vi "E7_20.vi"(4 "error in":T13, 7 "Command":T14) -> (0 "error out":T13, 3 "Response":T11)   [LabVIEW 2018]
uses:
  MOKO_LabViewLibrary/MokoLowLevel/MokoLowLovelControl/MLLC_Command.ctl
  MOKO_LabViewLibrary/MokoLowLevel/MokoLowLovelControl/MLLC_Error.ctl
  MOKO_LabViewLibrary/MokoLowLevel/MokoLowLovelControl/MLLC_Mode.ctl
  MOKO_LabViewLibrary/MokoLowLevel/MokoLowLovelControl/MLLC_Response.ctl
  MOKO_LabViewLibrary/MokoLowLevel/MokoLowLovelControl/MLLC_DriverName.ctl
  MOKO_LabViewLibrary/MokoLowLevel/MokoLowLovelControl/MLLC_ResponseInit.ctl
  MOKO_LabViewLibrary/MokoLowLevel/MokoLowLovelControl/MLLC_ErrorCode.ctl
  MOKO_LabViewLibrary/MokoLowLevel/MokoLowLovelControl/MLLC_Request.ctl
  MOKO_LabViewLibrary/MokoLowLevel/MokoLowLovelControl/MLLC_ConnectCluster.ctl
  MOKO_LabViewLibrary/MokoLowLevel/MokoLowLovelControl/MLLC_InterfaceType.ctl
  MOKO_LabViewLibrary/MokoLowLevel/MokoLowLovelControl/MLLC_OpenedSession.ctl
  MOKO_LabViewLibrary/MokoLowLevel/MokoLowLovelControl/MLLC_InterfaceSettings.ctl
  MOKO_LabViewLibrary/MokoLowLevel/MokoLowLovelControl/MLLC_InterfaceKind.ctl
  MOKO_LabViewLibrary/MokoLowLevel/MokoLowLovelControl/MLLC_Rs232Settings.ctl
panel:
  in  "Settings":T7={"Data"={"Connect"={"InterfaceType"=enum."VISA", "OpenedSession"="", "InterfaceSettings"={"Interface"=enum."RS232", "EOS 4 read"=enum."LF (\\n)", "EOS 4 write"=enum."LF (\\n)", "TMO, ms"=10000, "Sett"=variant(cluster{"Baud Rate":u32, "Data Bits":u16, "Parity":u16, "Stop Bits":u16, "Flow Control":u16, "Eho":bool} {"Baud Rate"=75, "Data Bits"=0, "Parity"=0, "Stop Bits"=0, "Flow Control"=0, "Eho"=FALSE})}}, "Function"=enum."VDC", "Delay, ms"=100}, "Saved Data"=variant}
  in  "Request":T8
  in  "Error Code":T6=5422
  in  "ResponseInit":T9="Є"
  in  "Driver Name":T10="E7_20"
  in  "Mode":T12=enum."Check"
  # "E7-20"
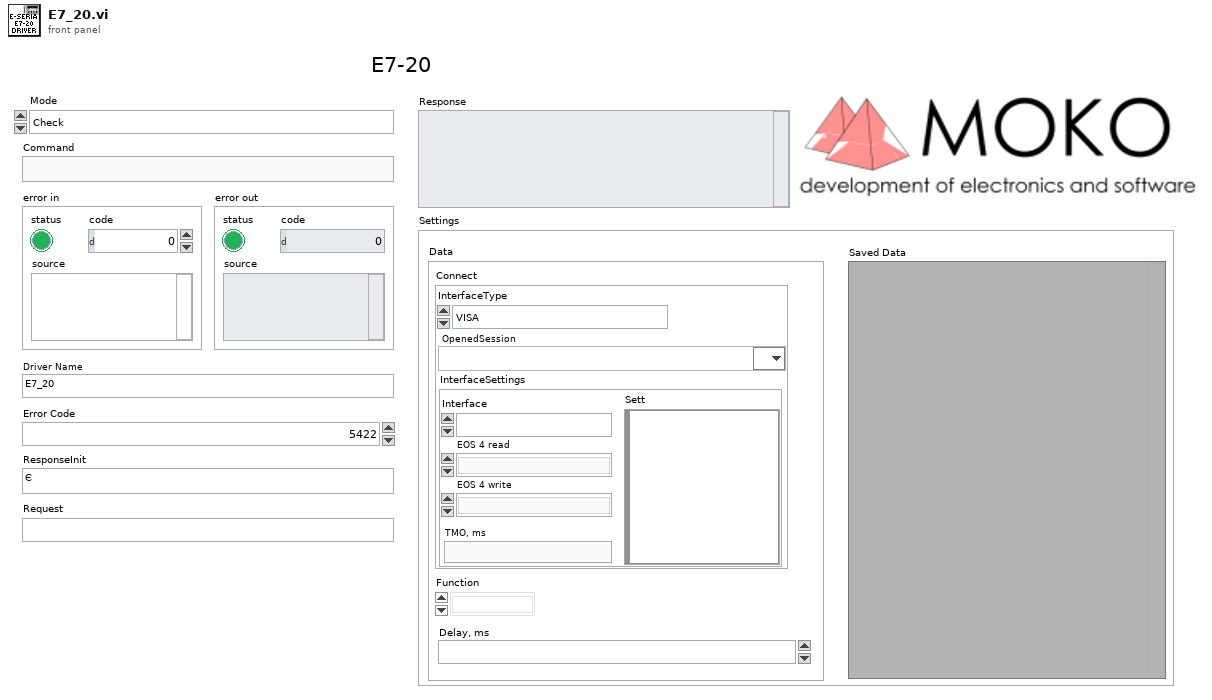
[diagram p1: front panel]
types:
  T1 = typedef "MLLC_ConnectCluster.ctl" = cluster{"InterfaceType":T2, "OpenedSession":T3, "InterfaceSettings":T4}
  T2 = typedef "MLLC_InterfaceType.ctl" = enum16{"VISA", "Prologix USB-GPIB"}
  T3 = typedef "MLLC_OpenedSession.ctl" = refnum<visa-resource-name>
  T4 = typedef "MLLC_InterfaceSettings.ctl" = cluster{"Interface":T5, "EOS 4 read":enum16{"Default (=EOS 4 write)", "CR (\\r)", "LF (\\n)", "None"}, "EOS 4 write":enum16{"CR+LF (\\r\\n)", "CR (\\r)", "LF (\\n)", "None"}, "TMO, ms":i32, "Sett":variant}
  T5 = typedef "MLLC_InterfaceKind.ctl" = enum16{"RS232", "GPIB", "USB", "Ethernet", "another"}
  T6 = typedef "MLLC_ErrorCode.ctl" = u32
  T7 = cluster{"Data":cluster{"Connect":T1, "Function":enum16{"F", "T", "R4", "R", "IAC", "IDC", "VAC", "VDC"}, "Delay, ms":T6}, "Saved Data":variant}
  T8 = typedef "MLLC_Request.ctl" = string
  T9 = typedef "MLLC_ResponseInit.ctl" = string
  T10 = typedef "MLLC_DriverName.ctl" = string
  T11 = typedef "MLLC_Response.ctl" = string
  T12 = typedef "MLLC_Mode.ctl" = enum16{"get", "set", "close", "Init", "Check"}
  T13 = typedef "MLLC_Error.ctl" = errorcluster
  T14 = typedef "MLLC_Command.ctl" = string
  T15 = cluster{"Connect":T1, "Function":enum16{"F", "T", "R4", "R", "IAC", "IDC", "VAC", "VDC"}, "Delay, ms":T6}
  T16 = typedef "MLLC_Rs232Settings.ctl" = cluster{"Baud Rate":u32, "Data Bits":u16, "Parity":u16, "Stop Bits":u16, "Flow Control":u16, "Eho":bool, "Address":dbl}
  T17 = enum16{"F", "T", "R4", "R", "IAC", "IDC", "VAC", "VDC"}
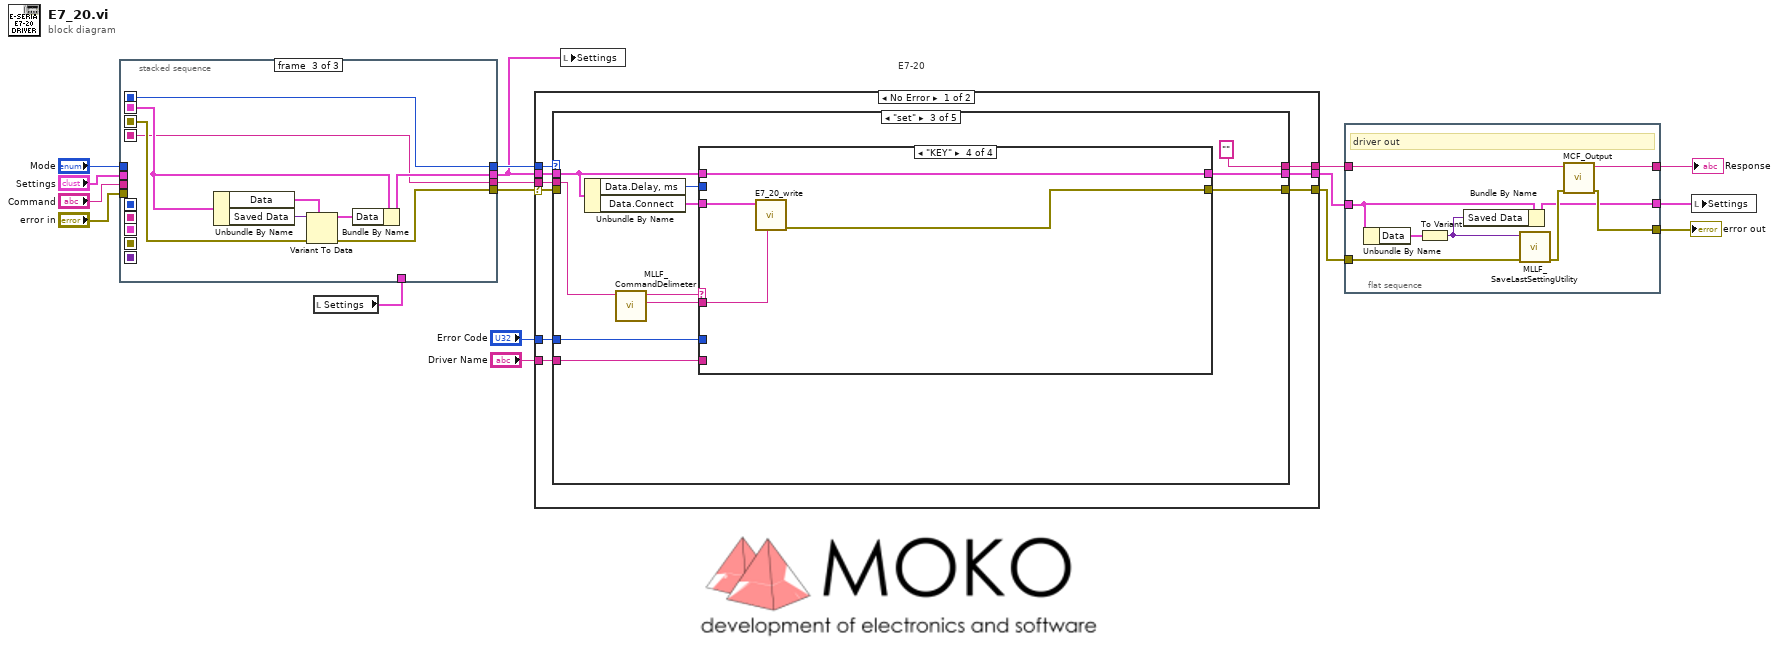
[diagram p0: block diagram]
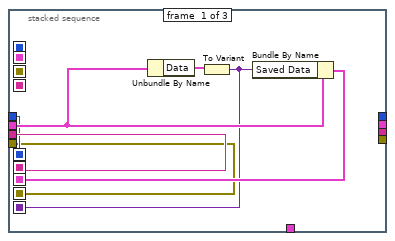
[diagram p2: hidden frame]
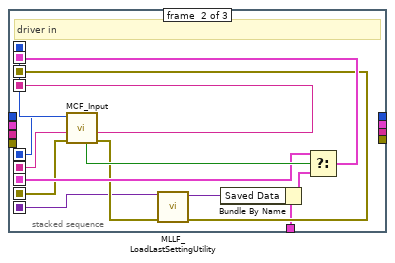
[diagram p3: hidden frame]
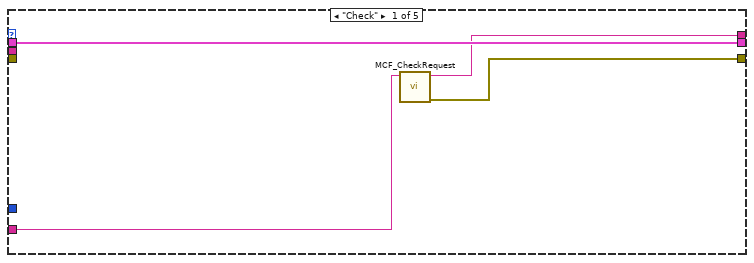
[diagram p4: hidden frame]
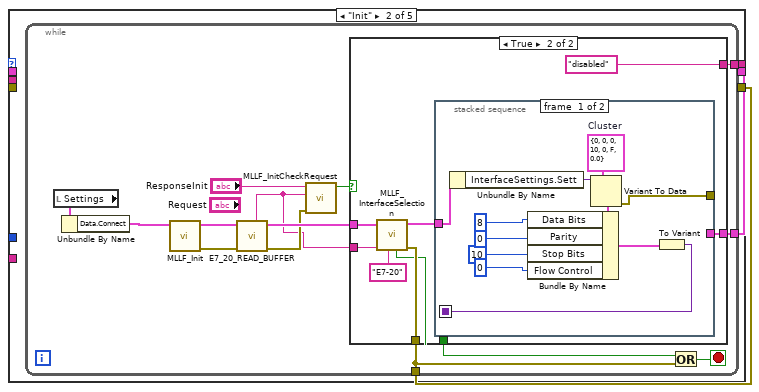
[diagram p5: hidden frame]
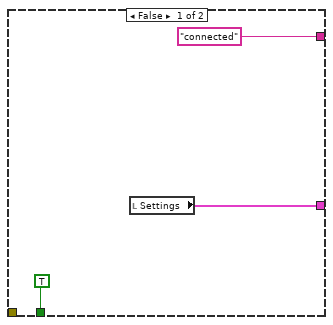
[diagram p6: hidden frame]
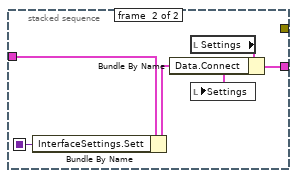
[diagram p7: hidden frame]
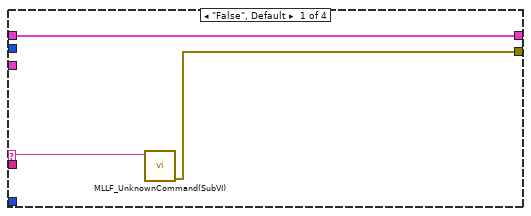
[diagram p8: hidden frame]
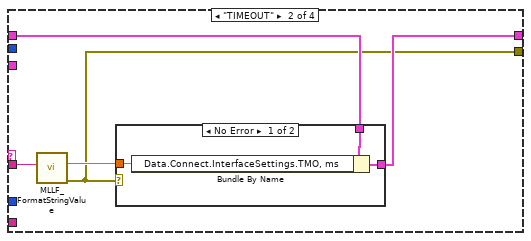
[diagram p9: hidden frame]
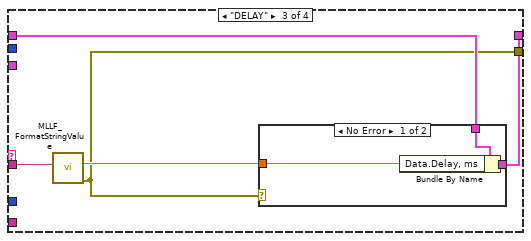
[diagram p11: hidden frame]
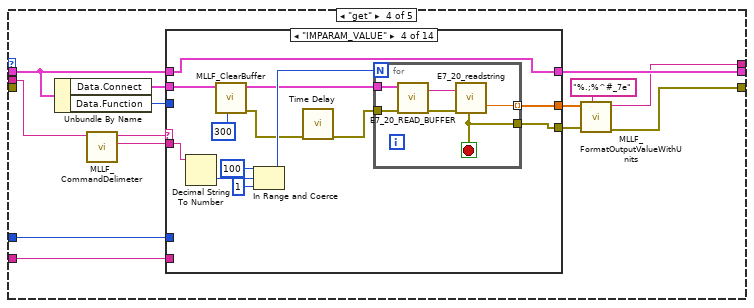
[diagram p13: hidden frame]
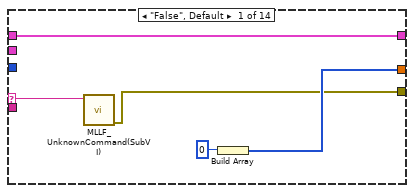
[diagram p14: hidden frame]
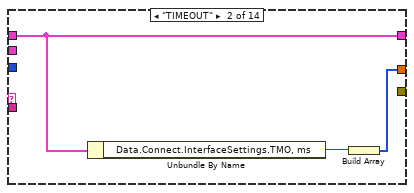
[diagram p15: hidden frame]
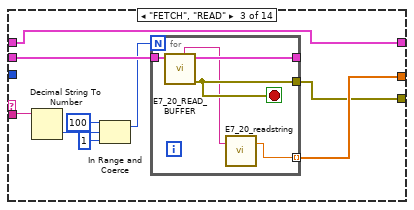
[diagram p16: hidden frame]
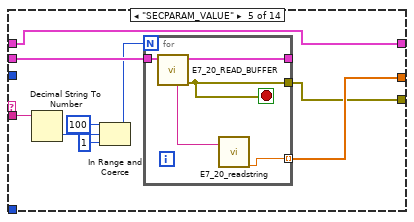
[diagram p17: hidden frame]
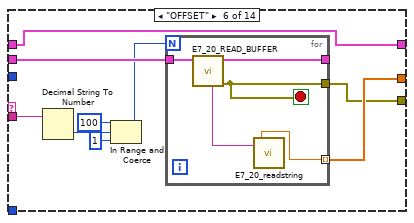
[diagram p18: hidden frame]
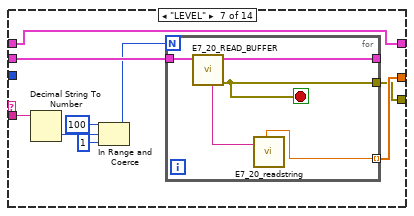
[diagram p19: hidden frame]
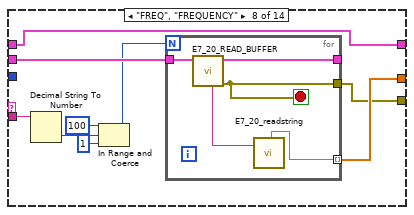
[diagram p20: hidden frame]
diagram:
  # "E7-20"
  n1 = local read "Settings"() -> (w7:T7)
  n2 = stacked-sequence {
    seq-local: [w20 _ _] -> [_ w36 _]
    seq-local: [w19 _ _] -> [_ w37 _]
    seq-local: [w22 _ _] -> [_ w32 _]
    seq-local: [w18 _ _] -> [_ w31 _]
    seq-local: [w21 _ _] -> [_ w27 _]
    seq-local: [_ w28 _] -> [_ _ w44]
    seq-local: [_ w38 _] -> [_ _ w41]
    seq-local: [_ w35 _] -> [_ _ w40]
    seq-local: [_ w34 _] -> [_ _ w45]
    tunnel: "Command" -> [w20 _ _]
    tunnel: "Mode" -> [w19 _ _]
    tunnel: "error in" -> [w18 _ _]
    tunnel: "Settings" -> [w23 _ _]
    tunnel: w7 -> [_ w26 _]
    tunnel: [_ _ w40] -> w9
    tunnel: [_ _ w43] -> w10
    tunnel: [_ _ w42] -> w8
    tunnel: [_ _ w41] -> w11
    frame #0 {
      n3 = Unbundle By Name(w23) -> ("Data"=w24:T15)
      n4 = To Variant(anything=w24) -> (Variant=w21:variant)
      n5 = Bundle By Name(cluster=w23, "Saved Data"=w21) -> (w22:T7)
    }
    frame #1 {
      # "driver in"
      n6 = call "MCF_Input.vi"("Error In"=w31, "Command in"=w36, "Mode in"=w37) -> ("Error Out"=w30:errorcluster, "Command out"=w35:string, "Mode out"=w38:T12, "Boolean"=w33:bool)  [unwired: 5 in]
      n7 = call "MLLF_LoadLastSettingUtility.vi"("Error In"=w30, "Save data in"=w27) -> ("Error Out"=w28:errorcluster, "Save data out"=w25:variant)  [unwired: 8 in]
      n8 = Bundle By Name(cluster=w26, "Saved Data"=w25) -> (w29:T7)
      n9 = Select(t=w32, s=w33, f=w29) -> (s? t:f=w34:T7)
    }
    frame #2 {
      n10 = Unbundle By Name(w45) -> ("Data"=w46:T15, "Saved Data"=w39:variant)
      n11 = Variant To Data(error in=w44, type=w46, Variant=w39) -> (data=w47:T15, error out=w42:errorcluster)
      n12 = Bundle By Name(cluster=w45, "Data"=w47) -> (w43:T7)
    }
  }
  n13 = case shown="No Error" w8 {
    selector: w8 -> [w52 w341]
    tunnel: [w54 w341] -> w4
    tunnel: w11 -> [w56 _]
    tunnel: [w55 "" ("String")] -> w6
    tunnel: w9 -> [w53 _]
    tunnel: w10 -> [w49 w340]
    tunnel: "Error Code" -> [w51 _]
    tunnel: "Driver Name" -> [w50 _]
    tunnel: [w48 w340] -> w5
    frame No Error {
      n14 = case shown="\"set\"" w56 {
        tunnel: [w59 w63 "" ("String") w141 _] -> w55
        tunnel: [w58 w61 w105 w142 w337] -> w54
        tunnel: w53 -> [_ _ w108 w145 _]
        tunnel: w52 -> [_ _ _ _ _]
        tunnel: w51 -> [_ _ w115 w152 _]
        tunnel: w50 -> [w57 _ w112 w151 _]
        tunnel: w49 -> [w60 _ w114 w154 w336]
        tunnel: [w60 w62 w113 w153 w336] -> w48
        frame "Check" {
          n15 = call "MCF_CheckRequest.vi"("Driver Name"=w57) -> ("Error Out"=w58:errorcluster, "Output String"=w59:string)  [unwired: 9 in]
        }
        frame "Init" {
          n16 = while {
            tunnel: [w75] -> w61
            tunnel: [w66] -> w63
            tunnel: [w65] -> w62
            stop <- w74 stop-if-true
            n17 = local read "Settings"() -> (w77:T7)
            n18 = Unbundle By Name(w77) -> ("Data.Connect"=w76:T1)
            n19 = call "MLLF_Init.vi"("DriverConnect in"=w76) -> ("Error Out"=w70:errorcluster, "DriverConnect out"=w71:T1)  [unwired: 7 in]
            n20 = call "E7_20_READ_BUFFER.vi"("error in"=w70, "DriverConnect in"=w71) -> ("error out"=w68:T13, "DriverConnect out"=w72:T1, "String"=w64:string)  [unwired: 7 in]
            n21 = call "MLLF_InitCheckRequest.vi"("error in (no error)"=w68, "Answer"=w64, "Response Init"="ResponseInit") -> ("Design"=w67:bool)  [unwired: 5 in, 3 out]
            n22 = case shown="True" w67 {
              tunnel: [_ w86] -> w75
              tunnel: [TRUE w82] -> w73
              tunnel: w72 -> [_ w88]
              tunnel: ["connected" "disabled"] -> w66
              tunnel: [w78 w83] -> w65
              tunnel: w64 -> [_ w81]
              frame False {
                n23 = local read "Settings"() -> (w78:T7)
              }
              frame True {
                n24 = call "MLLF_InterfaceSelection.vi"("Driver Name"="E7-20" ("String"), "Answer:"=w81, "DriverConnect in"=w88) -> ("error out"=w86:T13, "DriverConnect out"=w87:T1, "stop init?"=w82:bool)  [unwired: 4 in, 2 out]
                n25 = stacked-sequence {
                  seq-local: [w91 _] -> [_ w103]
                  tunnel: w87 -> [w89 w101]
                  tunnel: [w97 _] -> _
                  tunnel: [_ w102] -> w83
                  frame #0 {
                    w98 = T16 {"Baud Rate"=0, "Data Bits"=0, "Parity"=0, "Stop Bits"=10, "Flow Control"=0, "Eho"=FALSE, "Address"=0.0}  # Cluster
                    n26 = Unbundle By Name(w89) -> ("InterfaceSettings.Sett"=w99:variant)
                    n27 = Variant To Data(type=w98, Variant=w99) -> (data=w96:T16, error out=w97:errorcluster)  [unwired: 1 in]
                    n28 = Bundle By Name(cluster=w96, "Data Bits"=u16 8 ("Serial Settings:Data Bits"), "Parity"=u16 0 ("Serial Settings:Parity"), "Stop Bits"=u16 10 ("Serial Settings:Stop Bits"), "Flow Control"=u16 0 ("Serial Settings:Flow Control")) -> (w90:T16)
                    n29 = To Variant(anything=w90) -> (Variant=w91:variant)
                  }
                  frame #1 {
                    n30 = Bundle By Name(cluster=w101, "InterfaceSettings.Sett"=w103) -> (w100:T1)
                    n31 = local read "Settings"() -> (w104:T7)
                    n32 = Bundle By Name(cluster=w104, "Data.Connect"=w100) -> (w102:T7)
                    n33 = local write "Settings"(w102) -> ()
                  }
                }
              }
            }
            n34 = Or(x=w73, y=w75) -> (x .or. y?=w74:bool)
          }
        }
        frame "set" {
          n35 = Unbundle By Name(w114) -> ("Data.Delay, ms"=w109:T6, "Data.Connect"=w110:T1)
          n36 = call "MLLF_CommandDelimeter.vi"("command with param"=w108) -> ("param 1"=w106:string, "command"=w107:string)  [unwired: 6 in, 3 out]
          n37 = case shown="\"KEY\"" w107 {
            selector: w107 -> [w117 _ _ _]
            tunnel: w106 -> [_ w121 w130 w139]
            tunnel: [w116 w119 w128 w138] -> w105
            tunnel: w115 -> [_ _ _ _]
            tunnel: w114 -> [w118 w122 w131 w140]
            tunnel: [w118 w123 w132 w140] -> w113
            tunnel: w110 -> [_ _ _ w137]
            tunnel: w112 -> [_ _ _ _]
            tunnel: w109 -> [_ _ _ _]
            frame "False", Default {
              n38 = call "MLLF_UnknownCommand(SubVI).vi"("Unknown command"=w117) -> ("error out"=w116:errorcluster)  [unwired: 10 in]
            }
            frame "TIMEOUT" {
              n39 = call "MLLF_FormatStringValue.vi"("String Value"=w121) -> ("error out"=w119:T13, "number"=w120:dbl)  [unwired: 8 in, 1 out]
              n40 = case shown="No Error" w119 {
                tunnel: [w126 w127] -> w123
                tunnel: w122 -> [w125 w127]
                tunnel: w120 -> [w124 _]
                frame No Error {
                  n41 = Bundle By Name(cluster=w125, "Data.Connect.InterfaceSettings.TMO, ms"=w124) -> (w126:T7)
                }
                frame Error {
                }
              }
            }
            frame "DELAY" {
              n42 = call "MLLF_FormatStringValue.vi"("String Value"=w130) -> ("error out"=w128:T13, "number"=w129:dbl)  [unwired: 8 in, 1 out]
              n43 = case shown="No Error" w128 {
                tunnel: [w135 w136] -> w132
                tunnel: w131 -> [w134 w136]
                tunnel: w129 -> [w133 _]
                frame No Error {
                  n44 = Bundle By Name(cluster=w134, "Data.Delay, ms"=w133) -> (w135:T7)
                }
                frame Error {
                }
              }
            }
            frame "KEY" {
              n45 = call "E7_20_write.vi"("Command"=w139, "DriverConnect in"=w137) -> ("error out"=w138:T13)  [unwired: 8 in, 1 out]
            }
          }
        }
        frame "get" {
          n46 = Unbundle By Name(w154) -> ("Data.Connect"=w148:T1, "Data.Function"=w146:T17)
          n47 = call "MLLF_CommandDelimeter.vi"("command with param"=w145) -> ("param 1"=w143:string, "command"=w144:string)  [unwired: 6 in, 3 out]
          n48 = case shown="\"IMPARAM_VALUE\"" w144 {
            selector: w144 -> [w156 _ _ _ _ _ _ _ _ _ _ _ _ _]
            tunnel: w143 -> [_ _ w163 w177 w196 w210 w224 w238 w252 w266 w280 w294 w308 w322]
            tunnel: [w155 _ w168 w187 w201 w215 w229 w243 w257 w271 w285 w299 w313 w327] -> w150
            tunnel: w152 -> [_ _ _ _ _ _ _ _ _ _ _ _ _ _]
            tunnel: [w159 w162 w171 w189 w204 w218 w232 w246 w260 w274 w288 w302 w316 w330] -> w153
            tunnel: w154 -> [w159 w162 w171 w189 w204 w218 w232 w246 w260 w274 w288 w302 w316 w330]
            tunnel: [w157 w160 w169 w188 w202 w216 w230 w244 w258 w272 w286 w300 w314 w328] -> w149
            tunnel: w148 -> [_ _ w170 w180 w203 w217 w231 w245 w259 w273 w287 w301 w315 w329]
            tunnel: w151 -> [_ _ _ _ _ _ _ _ _ _ _ _ _ _]
            tunnel: w146 -> [_ _ _ _ _ _ _ _ _ _ _ _ _ _]
            frame "False", Default {
              n49 = call "MLLF_UnknownCommand(SubVI).vi"("Unknown command"=w156) -> ("error out"=w155:errorcluster)  [unwired: 10 in]
              n50 = Build Array(0 ("TimeOut")) -> (w157:i32[])
            }
            frame "TIMEOUT" {
              n51 = Unbundle By Name(w162) -> ("Data.Connect.InterfaceSettings.TMO, ms"=w161:i32)
              n52 = Build Array(w161) -> (w160:i32[])
            }
            frame "FETCH", "READ" {
              n53 = Decimal String To Number(string=w163) -> (number=w167:i32)  [unwired: 2 in, 1 out]
              n54 = In Range and Coerce(upper limit=100, x=w167, lower limit=1) -> (coerced(x)=w164:i32)  [unwired: 1 out]
              n55 = for {
                N: w164 -> [_]
                tunnel: [w172] -> w169 mode=indexing
                tunnel: [w175] -> w168
                tunnel: [w176] -> _
                tunnel: w170 -> [w174]
                stop <- w175 stop-if-true
                n56 = call "E7_20_READ_BUFFER.vi"("DriverConnect in"=w174) -> ("error out"=w175:T13, "DriverConnect out"=w176:T1, "String"=w173:string)  [unwired: 8 in]
                n57 = call "E7_20_readstring.vi"("read buffer"=w173) -> ("CS"=w172:dbl)  [unwired: 6 in, 12 out]
              }
            }
            frame "IMPARAM_VALUE" {
              n58 = Decimal String To Number(string=w177) -> (number=w186:i32)  [unwired: 2 in, 1 out]
              n59 = call "MLLF_ClearBuffer.vi"("Timeout(default = 300 ms)"=u32 300 ("Timeout"), "DriverConnect in"=w180) -> ("Error Out"=w179:errorcluster, "DriverConnect out"=w181:T1)  [unwired: 6 in, 1 out]
              n60 = In Range and Coerce(upper limit=100, x=w186, lower limit=1) -> (coerced(x)=w183:i32)  [unwired: 1 out]
              n61 = call "Time Delay"("error in (no error)"=w179) -> ("error out"=w178:errorcluster)  [unwired: 10 in]
              n62 = for {
                N: w183 -> [_]
                tunnel: [w193] -> w188 mode=indexing
                tunnel: [w191] -> w187
                tunnel: w181 -> [w194]
                tunnel: w178 -> [w190]
                stop <- w191 stop-if-true
                n63 = call "E7_20_READ_BUFFER.vi"("error in"=w190, "DriverConnect in"=w194) -> ("error out"=w192:T13, "String"=w195:string)  [unwired: 7 in, 1 out]
                n64 = call "E7_20_readstring.vi"("read buffer"=w195, "Error In"=w192) -> ("Error Out"=w191:errorcluster, "ImParam_Value"=w193:dbl)  [unwired: 5 in, 11 out]
              }
            }
            frame "SECPARAM_VALUE" {
              n65 = Decimal String To Number(string=w196) -> (number=w200:i32)  [unwired: 2 in, 1 out]
              n66 = In Range and Coerce(upper limit=100, x=w200, lower limit=1) -> (coerced(x)=w197:i32)  [unwired: 1 out]
              n67 = for {
                N: w197 -> [_]
                tunnel: [w205] -> w202 mode=indexing
                tunnel: [w208] -> w201
                tunnel: [w209] -> _
                tunnel: w203 -> [w206]
                stop <- w208 stop-if-true
                n68 = call "E7_20_READ_BUFFER.vi"("DriverConnect in"=w206) -> ("error out"=w208:T13, "DriverConnect out"=w209:T1, "String"=w207:string)  [unwired: 8 in]
                n69 = call "E7_20_readstring.vi"("read buffer"=w207) -> ("SecParam_Value"=w205:dbl)  [unwired: 6 in, 12 out]
              }
            }
            frame "OFFSET" {
              n70 = Decimal String To Number(string=w210) -> (number=w214:i32)  [unwired: 2 in, 1 out]
              n71 = In Range and Coerce(upper limit=100, x=w214, lower limit=1) -> (coerced(x)=w211:i32)  [unwired: 1 out]
              n72 = for {
                N: w211 -> [_]
                tunnel: [w219] -> w216 mode=indexing
                tunnel: [w222] -> w215
                tunnel: [w223] -> _
                tunnel: w217 -> [w220]
                stop <- w222 stop-if-true
                n73 = call "E7_20_READ_BUFFER.vi"("DriverConnect in"=w220) -> ("error out"=w222:T13, "DriverConnect out"=w223:T1, "String"=w221:string)  [unwired: 8 in]
                n74 = call "E7_20_readstring.vi"("read buffer"=w221) -> ("Offset"=w219:dbl)  [unwired: 6 in, 12 out]
              }
            }
            frame "LEVEL" {
              n75 = Decimal String To Number(string=w224) -> (number=w228:i32)  [unwired: 2 in, 1 out]
              n76 = In Range and Coerce(upper limit=100, x=w228, lower limit=1) -> (coerced(x)=w225:i32)  [unwired: 1 out]
              n77 = for {
                N: w225 -> [_]
                tunnel: [w233] -> w230 mode=indexing
                tunnel: [w236] -> w229
                tunnel: [w237] -> _
                tunnel: w231 -> [w234]
                stop <- w236 stop-if-true
                n78 = call "E7_20_READ_BUFFER.vi"("DriverConnect in"=w234) -> ("error out"=w236:T13, "DriverConnect out"=w237:T1, "String"=w235:string)  [unwired: 8 in]
                n79 = call "E7_20_readstring.vi"("read buffer"=w235) -> ("Level"=w233:dbl)  [unwired: 6 in, 12 out]
              }
            }
            frame "FREQ", "FREQUENCY" {
              n80 = Decimal String To Number(string=w238) -> (number=w242:i32)  [unwired: 2 in, 1 out]
              n81 = In Range and Coerce(upper limit=100, x=w242, lower limit=1) -> (coerced(x)=w239:i32)  [unwired: 1 out]
              n82 = for {
                N: w239 -> [_]
                tunnel: [w247] -> w244 mode=indexing
                tunnel: [w250] -> w243
                tunnel: [w251] -> _
                tunnel: w245 -> [w248]
                stop <- w250 stop-if-true
                n83 = call "E7_20_READ_BUFFER.vi"("DriverConnect in"=w248) -> ("error out"=w250:T13, "DriverConnect out"=w251:T1, "String"=w249:string)  [unwired: 8 in]
                n84 = call "E7_20_readstring.vi"("read buffer"=w249) -> ("Frequency"=w247:dbl)  [unwired: 6 in, 12 out]
              }
            }
            frame "FLAGS" {
              n85 = Decimal String To Number(string=w252) -> (number=w256:i32)  [unwired: 2 in, 1 out]
              n86 = In Range and Coerce(upper limit=100, x=w256, lower limit=1) -> (coerced(x)=w253:i32)  [unwired: 1 out]
              n87 = for {
                N: w253 -> [_]
                tunnel: [w261] -> w258 mode=indexing
                tunnel: [w264] -> w257
                tunnel: [w265] -> _
                tunnel: w259 -> [w262]
                stop <- w264 stop-if-true
                n88 = call "E7_20_READ_BUFFER.vi"("DriverConnect in"=w262) -> ("error out"=w264:T13, "DriverConnect out"=w265:T1, "String"=w263:string)  [unwired: 8 in]
                n89 = call "E7_20_readstring.vi"("read buffer"=w263) -> ("FLAGS"=w261:dbl)  [unwired: 6 in, 12 out]
              }
            }
            frame "MODE" {
              n90 = Decimal String To Number(string=w266) -> (number=w270:i32)  [unwired: 2 in, 1 out]
              n91 = In Range and Coerce(upper limit=100, x=w270, lower limit=1) -> (coerced(x)=w267:i32)  [unwired: 1 out]
              n92 = for {
                N: w267 -> [_]
                tunnel: [w275] -> w272 mode=indexing
                tunnel: [w278] -> w271
                tunnel: [w279] -> _
                tunnel: w273 -> [w276]
                stop <- w278 stop-if-true
                n93 = call "E7_20_READ_BUFFER.vi"("DriverConnect in"=w276) -> ("error out"=w278:T13, "DriverConnect out"=w279:T1, "String"=w277:string)  [unwired: 8 in]
                n94 = call "E7_20_readstring.vi"("read buffer"=w277) -> ("Mode"=w275:dbl)  [unwired: 6 in, 12 out]
              }
            }
            frame "LIMIT" {
              n95 = Decimal String To Number(string=w280) -> (number=w284:i32)  [unwired: 2 in, 1 out]
              n96 = In Range and Coerce(upper limit=100, x=w284, lower limit=1) -> (coerced(x)=w281:i32)  [unwired: 1 out]
              n97 = for {
                N: w281 -> [_]
                tunnel: [w289] -> w286 mode=indexing
                tunnel: [w292] -> w285
                tunnel: [w293] -> _
                tunnel: w287 -> [w290]
                stop <- w292 stop-if-true
                n98 = call "E7_20_READ_BUFFER.vi"("DriverConnect in"=w290) -> ("error out"=w292:T13, "DriverConnect out"=w293:T1, "String"=w291:string)  [unwired: 8 in]
                n99 = call "E7_20_readstring.vi"("read buffer"=w291) -> ("Limit"=w289:dbl)  [unwired: 6 in, 12 out]
              }
            }
            frame "IMPARAM" {
              n100 = Decimal String To Number(string=w294) -> (number=w298:i32)  [unwired: 2 in, 1 out]
              n101 = In Range and Coerce(upper limit=100, x=w298, lower limit=1) -> (coerced(x)=w295:i32)  [unwired: 1 out]
              n102 = for {
                N: w295 -> [_]
                tunnel: [w303] -> w300 mode=indexing
                tunnel: [w306] -> w299
                tunnel: [w307] -> _
                tunnel: w301 -> [w304]
                stop <- w306 stop-if-true
                n103 = call "E7_20_READ_BUFFER.vi"("DriverConnect in"=w304) -> ("error out"=w306:T13, "DriverConnect out"=w307:T1, "String"=w305:string)  [unwired: 8 in]
                n104 = call "E7_20_readstring.vi"("read buffer"=w305) -> ("ImParam"=w303:dbl)  [unwired: 6 in, 12 out]
              }
            }
            frame "SECPARAM" {
              n105 = Decimal String To Number(string=w308) -> (number=w312:i32)  [unwired: 2 in, 1 out]
              n106 = In Range and Coerce(upper limit=100, x=w312, lower limit=1) -> (coerced(x)=w309:i32)  [unwired: 1 out]
              n107 = for {
                N: w309 -> [_]
                tunnel: [w317] -> w314 mode=indexing
                tunnel: [w320] -> w313
                tunnel: [w321] -> _
                tunnel: w315 -> [w318]
                stop <- w320 stop-if-true
                n108 = call "E7_20_READ_BUFFER.vi"("DriverConnect in"=w318) -> ("error out"=w320:T13, "DriverConnect out"=w321:T1, "String"=w319:string)  [unwired: 8 in]
                n109 = call "E7_20_readstring.vi"("read buffer"=w319) -> ("SecParam"=w317:dbl)  [unwired: 6 in, 12 out]
              }
            }
            frame "ONCHANGE" {
              n110 = Decimal String To Number(string=w322) -> (number=w326:i32)  [unwired: 2 in, 1 out]
              n111 = In Range and Coerce(upper limit=100, x=w326, lower limit=1) -> (coerced(x)=w323:i32)  [unwired: 1 out]
              n112 = for {
                N: w323 -> [_]
                tunnel: [w331] -> w328 mode=indexing
                tunnel: [w334] -> w327
                tunnel: [w335] -> _
                tunnel: w329 -> [w332]
                stop <- w334 stop-if-true
                n113 = call "E7_20_READ_BUFFER.vi"("DriverConnect in"=w332) -> ("error out"=w334:T13, "DriverConnect out"=w335:T1, "String"=w333:string)  [unwired: 8 in]
                n114 = call "E7_20_readstring.vi"("read buffer"=w333) -> ("OnChange"=w331:dbl)  [unwired: 6 in, 12 out]
              }
            }
          }
          n115 = call "MLLF_FormatOutputValueWithUnits.vi"("Format"="%.;%^#_7e" ("format string"), "error in"=w150, "ValuesIn"=w149) -> ("error out"=w142:T13, "Result string"=w141:T14)  [unwired: 7 in]
        }
        frame "close" {
          n116 = Unbundle By Name(w336) -> ("Data.Connect.OpenedSession"=w338:T3)
          n117 = VISA Close(VISA resource name=w338) -> (error out=w337:errorcluster)  [unwired: 1 in]
        }
      }
    }
    frame Error {
    }
  }
  n118 = local write "Settings"(w10) -> ()
  n119 = flat-sequence {
    tunnel: [w350] -> w3
    tunnel: [w349] -> w1
    tunnel: w6 -> [w348]
    tunnel: w4 -> [w347]
    tunnel: w5 -> [w343]
    tunnel: [w345] -> w2
    frame #0 {
      # "driver out"
      n120 = Unbundle By Name(w343) -> ("Data"=w342:T15)
      n121 = To Variant(anything=w342) -> (Variant=w344:variant)
      n122 = Bundle By Name(cluster=w343, "Saved Data"=w344) -> (w345:T7)
      n123 = call "MLLF_SaveLastSettingUtility.vi"("error in"=w347, "Saved Data"=w344) -> ("error out"=w346:T13)  [unwired: 8 in, 1 out]
      n124 = call "MCF_Output.vi"("Error In"=w346, "Input"=w348) -> ("Error Out"=w349:errorcluster, "Output"=w350:string)  [unwired: 8 in]
    }
  }
  n125 = local write "Settings"(w2) -> ()
  "error out" <- w1
  "Response" <- w3
